vi "Kalman filter - Angle 1st (SubVI).vi"(1 "Bias":dbl, 2 "Gyroscope":dbl, 3 "dt":dbl, 4 "Angle in":dbl) -> (0 "Angle out":dbl)   [LabVIEW 2013]
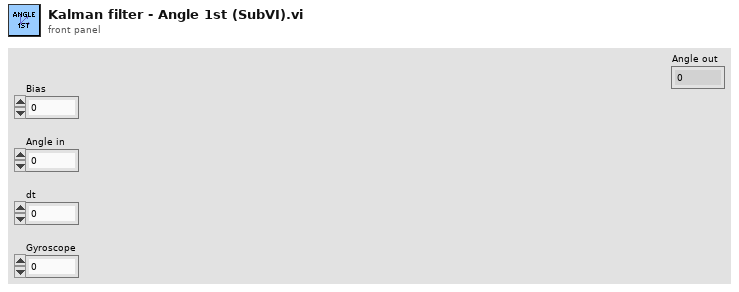
[diagram p1: front panel]
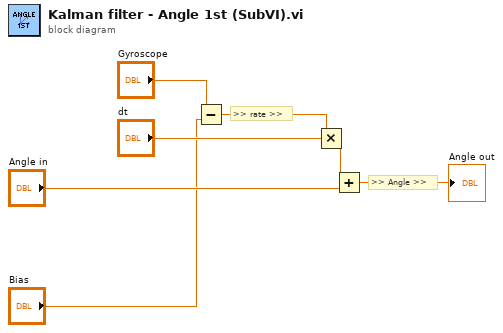
[diagram p0: block diagram]
diagram:
  # ">> Angle >>"
  # ">> rate >>"
  n1 = Subtract(x="Gyroscope", y="Bias") -> (x-y=w6:dbl)
  n2 = Multiply(x=w6, y="dt") -> (x*y=w5:dbl)
  n3 = Add(x=w5, y="Angle in") -> (x+y=→"Angle out":dbl)
